vi "Set Data.vi"(6 "DIO ref":refnum<vi>, 9 "NInput":i32, 11 "Data":T1) -> (3 "Data out":T1)   [LabVIEW 2015, in "Digital I-O.xctl"]
uses:
  Digital I-O.xctl
  Data.ctl
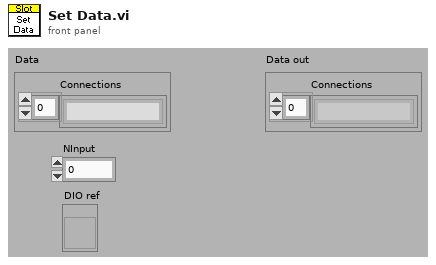
[diagram p1: front panel]
types:
  T1 = typedef "Digital I-O.xctl/Data.ctl" = cluster{"Connections":string[]}
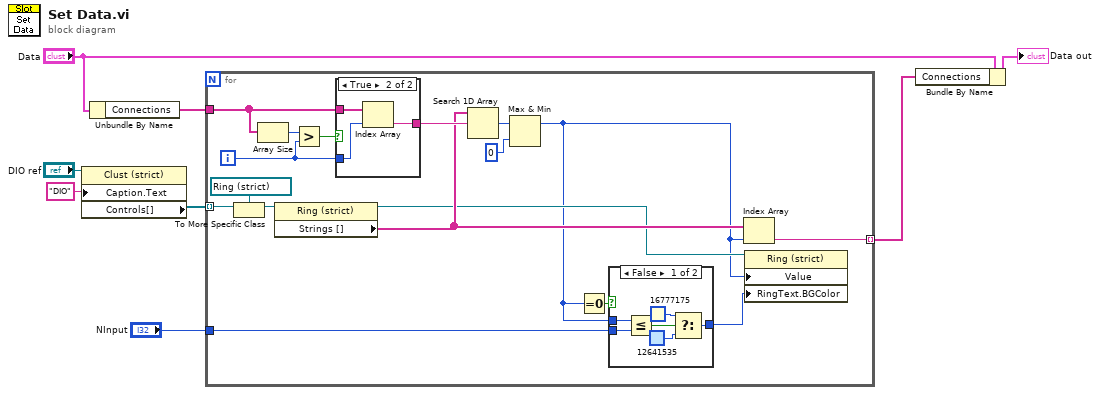
[diagram p0: block diagram]
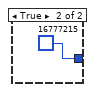
[diagram p2: hidden frame]
diagram:
  n1 = property class="Clust (strict)"(reference="DIO ref", "Caption.Text"="DIO") -> ("Controls[]"=w3:refnum<vi>[])  [unwired: 1 in, 2 out]
  n2 = Unbundle By Name("Data") -> ("Connections"=w6:string[])
  n3 = for {
    tunnel: w6 -> [w23]
    tunnel: w3 -> [w21] mode=indexing
    tunnel: [w16] -> w5 mode=indexing
    tunnel: "NInput" -> [w10]
    i -> [w22]
    n4 = To More Specific Class(target class=refnum<vi> refnum ("Ring 2"), reference=w21) -> (specific class reference=w14:refnum<vi>)  [unwired: 1 in, 1 out]
    n5 = Array Size(array=w23) -> (size(s)=w25:i32)
    n6 = property class="Ring (strict)"(reference=w14) -> (reference out=w15:refnum<vi>, "Strings []"=w17:string[])  [unwired: 1 in, 1 out]
    n7 = Greater?(x=w25, y=w22) -> (0:w24:bool)
    n8 = case shown="True" w24 {
      tunnel: w23 -> [_ w35]
      tunnel: w22 -> [_ w34]
      tunnel: [_ w33] -> w18
      frame False {
      }
      frame True {
        n9 = Index Array(array=w35, index=w34) -> (element=w33:string)
      }
    }
    n10 = Search 1D Array(1D array=w17, element=w18) -> (index of element=w19:i32)  [unwired: 1 in]
    n11 = Max & Min(x=w19, y=0) -> (max(x,y)=w9:i32)  [unwired: 1 out]
    n12 = Equal To 0?(x=w9) -> (x = 0?=w12:bool)
    n13 = case shown="False" w12 {
      tunnel: w9 -> [w31 _]
      tunnel: w10 -> [w30 _]
      tunnel: [w26 u32 16777215] -> w11
      frame False {
        n14 = Less Or Equal?(x=w31, y=w30) -> (x <= y?=w29:bool)
        n15 = Select(t=u32 16777175, s=w29, f=u32 12641535) -> (s? t:f=w26:u32)
      }
      frame True {
      }
    }
    n16 = Index Array(array=w17, index=w9) -> (element=w16:string)
    n17 = property class="Ring (strict)"(reference=w15, "Value"=w9, "RingText.BGColor"=w11) -> ()  [unwired: 1 in, 2 out]
  }
  n18 = Bundle By Name(cluster="Data", "Connections"=w5) -> (→"Data out":T1)
